vi "BLM Control Text Out.vi"(1 "BLM Control":T2={"extra wait"=0, "Stepper Value"=1e-09, "Value 1"=1.0, "Value 2"=1.0, "String 1"="", "String 2"=""} {"Value 2" format="%#_6e"; "Value 1" format="%<%H:%M:%S>t"; "extra wait" min=0; "Stepper Value" step=0.045 format="%#.7e"}) -> (0 "Command text":string[][](array[string]))   [LabVIEW 2021]
uses:
  BLM Control.ctl
panel:
  out "Est Time (H:M:S)":dbl
  out "Top or Bottom":T1(ring)
  out "String Cluster":T3
  # "BLM (Brushless Motor) Control"
  # "(BLM_ManualControl.vi needs to be open before using this program)"
  # "Distance:"
  # "deg of BLM:"
  # "seconds"
  # "AND wait extra"
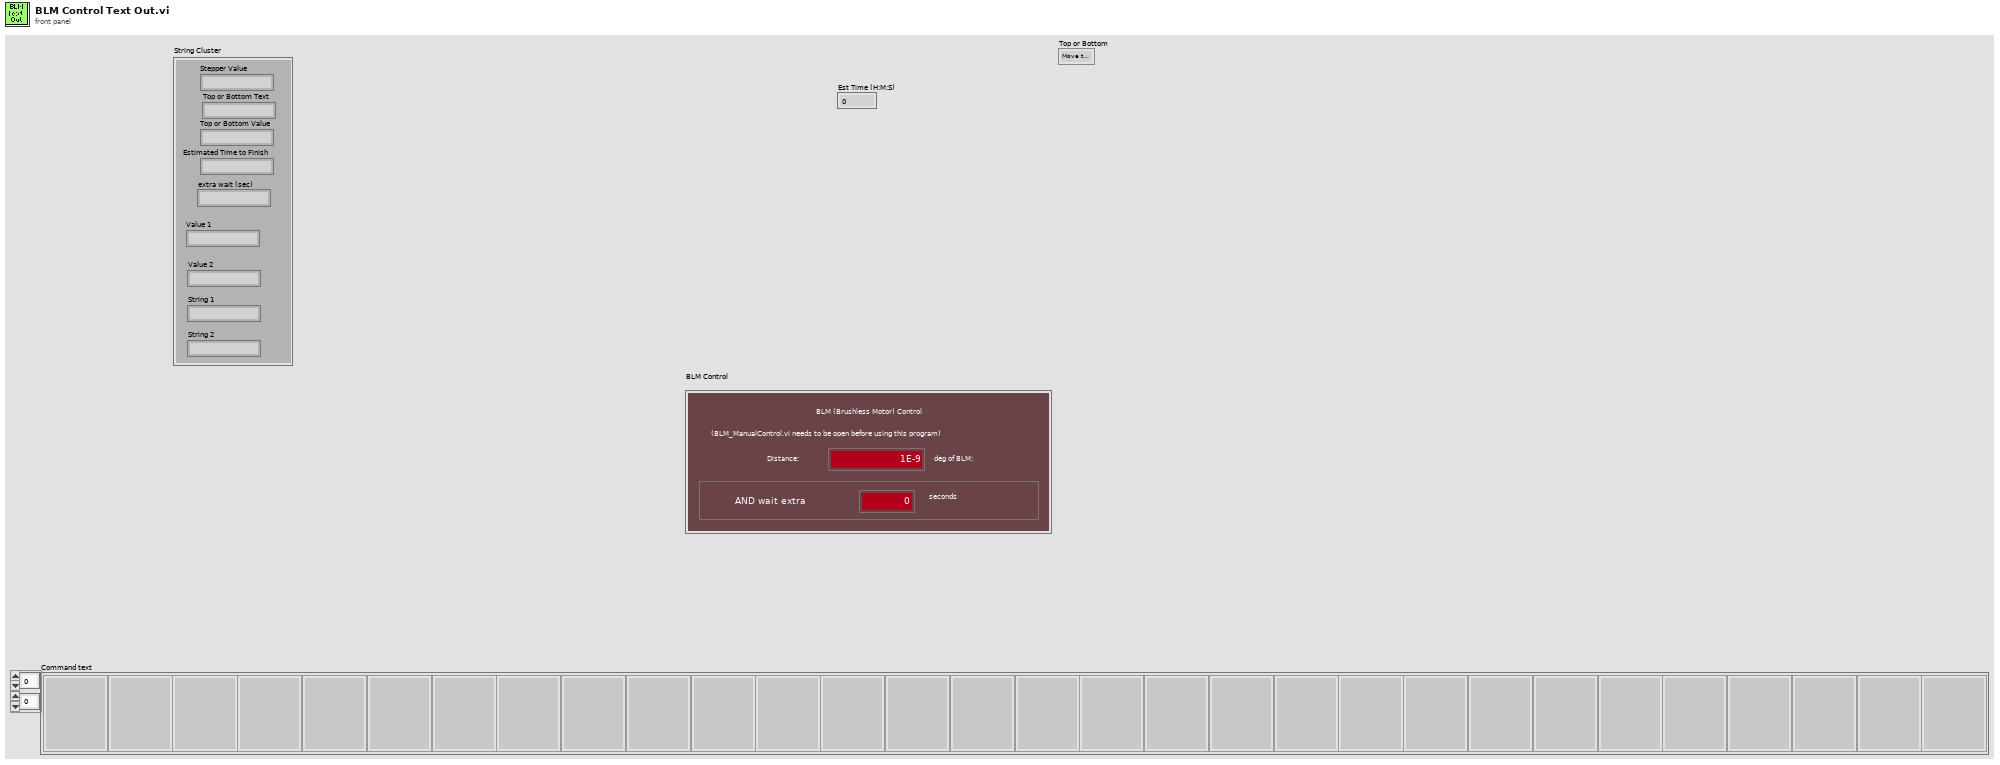
[diagram p1: front panel]
types:
  T1 = enum32{"Move to Top Position (deg)", "Move to Bottom Position (deg or in)"}
  T2 = typedef "BLM Control.ctl" = cluster{"extra wait":i32, "Stepper Value":dbl, "Value 1":dbl, "Value 2":dbl, "String 1":string, "String 2":string}
  T3 = cluster{"Stepper Value":string, "Top or Bottom Value":string, "Estimated Time to Finish":string, "extra wait (sec)":string, "Top or Bottom Text":string, "Value 1":string, "Value 2":string, "String 1":string, "String 2":string}
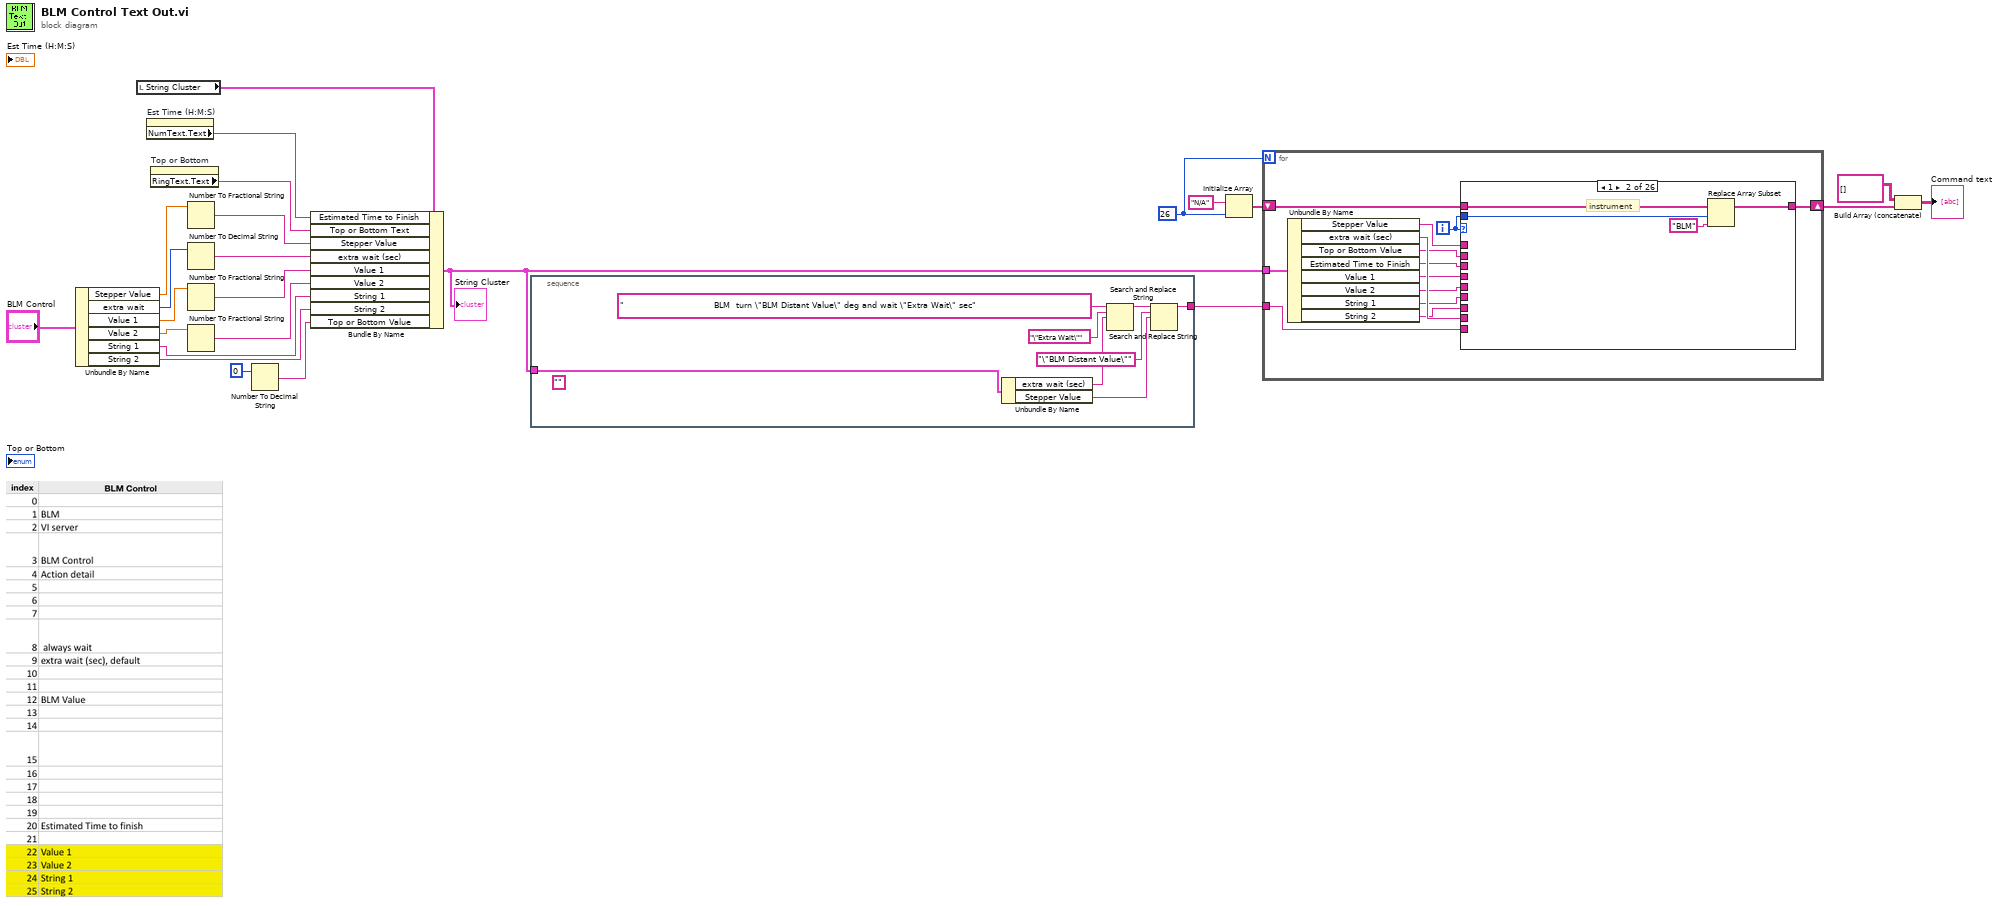
[diagram p0: block diagram]
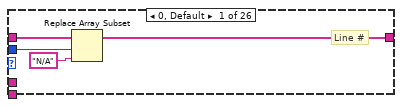
[diagram p2: hidden frame]
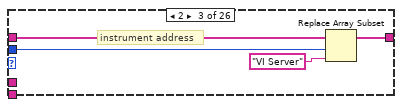
[diagram p3: hidden frame]
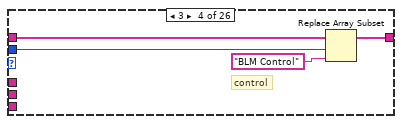
[diagram p4: hidden frame]
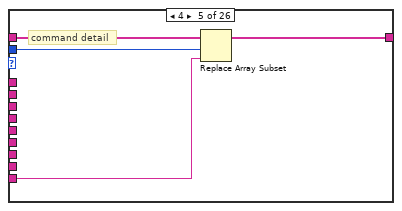
[diagram p5: hidden frame]
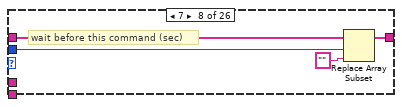
[diagram p8: hidden frame]
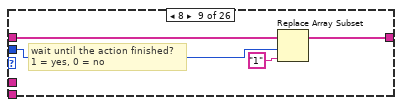
[diagram p9: hidden frame]
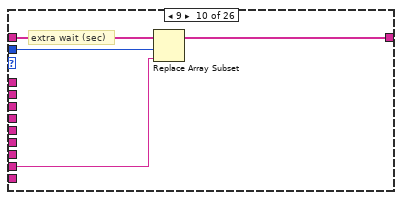
[diagram p10: hidden frame]
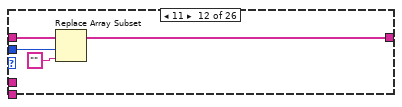
[diagram p12: hidden frame]
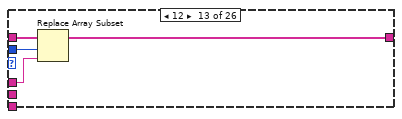
[diagram p13: hidden frame]
diagram:
  w21 = 26
  n1 = Unbundle By Name("BLM Control") -> ("Stepper Value"=w5:dbl, "extra wait"=w14:i32, "Value 1"=w12:dbl, "Value 2"=w11:dbl, "String 1"=w8:string, "String 2"=w7:string)
  n2 = local read "String Cluster"() -> (w18:T3)
  n3 = property on="Est Time (H:M:S)" class="DigNum (strict)"() -> ("NumText.Text"=w3:string)  [unwired: 2 in, 2 out]
  n4 = property on="Top or Bottom" class="Enum (strict)"() -> ("RingText.Text"=w6:string)  [unwired: 2 in, 2 out]
  n5 = Number To Fractional String(number=w5) -> (F-format string=w4:string)  [unwired: 3 in]
  n6 = Number To Decimal String(number=w14) -> (decimal integer string=w13:string)  [unwired: 1 in]
  n7 = Number To Fractional String(number=w12) -> (F-format string=w10:string)  [unwired: 3 in]
  n8 = Number To Fractional String(number=w11) -> (F-format string=w9:string)  [unwired: 3 in]
  n9 = Number To Decimal String(number=0) -> (decimal integer string=w2:string)  [unwired: 1 in]
  n10 = Bundle By Name(cluster=w18, "Estimated Time to Finish"=w3, "Top or Bottom Text"=w6, "Stepper Value"=w4, "extra wait (sec)"=w13, "Value 1"=w10, "Value 2"=w9, "String 1"=w8, "String 2"=w7, "Top or Bottom Value"=w2) -> (w16:T3)
  "String Cluster" <- w16
  n11 = stacked-sequence {
    tunnel: [w25] -> w17
    tunnel: w16 -> [w28]
    frame #0 {
      (unwired) "" ("search string")
      n12 = Unbundle By Name(w28) -> ("extra wait (sec)"=w27:string, "Stepper Value"=w26:string)
      n13 = Search and Replace String(input string="                              BLM  turn \"BLM Distant Value\" deg and wait \"Extra Wait\" sec", search string="\"Extra Wait\"", replace string=w27) -> (result string=w32:string)  [unwired: 5 in, 3 out]
      n14 = Search and Replace String(input string=w32, search string="\"BLM Distant Value\"", replace string=w26) -> (result string=w25:string)  [unwired: 5 in, 3 out]
    }
  }
  n15 = Initialize Array("N/A", w21) -> (w20:string[])
  n16 = for {
    N: w21 -> [_]
    shift-right: [w43] -> w19
    shift-left: w20 -> [w44]
    tunnel: w17 -> [w42]
    tunnel: w16 -> [w41]
    i -> [w45]
    n17 = Unbundle By Name(w41) -> ("Stepper Value"=w40:string, "extra wait (sec)"=w39:string, "Top or Bottom Value"=w34:string, "Estimated Time to Finish"=w33:string, "Value 1"=w38:string, "Value 2"=w37:string, "String 1"=w36:string, "String 2"=w35:string)
    n18 = case shown="1" w45 {
      tunnel: w45 -> [w48 w52 w57 w59 w64 _ _ w69 w73 w77 _ w82 w86 _ _ _ _ _ _ _ w97 _ w101 w106 w110 w114]
      tunnel: w44 -> [w49 w51 w56 w60 w65 w66 w67 w71 w75 w79 w80 w83 w88 w89 w90 w91 w92 w93 w94 w95 w99 w100 w103 w108 w112 w115]
      tunnel: [w46 w50 w55 w58 w63 w66 w67 w70 w74 w78 w80 w84 w87 w89 w90 w91 w92 w93 w94 w95 w98 w100 w102 w107 w111 w116] -> w43
      tunnel: w42 -> [_ _ _ _ w62 _ _ _ _ _ _ _ _ _ _ _ _ _ _ _ _ _ _ _ _ _]
      tunnel: w40 -> [_ _ _ _ _ _ _ _ _ _ _ _ w85 _ _ _ _ _ _ _ _ _ _ _ _ _]
      tunnel: w39 -> [_ _ _ _ _ _ _ _ _ w76 _ _ _ _ _ _ _ _ _ _ _ _ _ _ _ _]
      tunnel: w38 -> [_ _ _ _ _ _ _ _ _ _ _ _ _ _ _ _ _ _ _ _ _ _ w104 _ _ _]
      tunnel: w37 -> [_ _ _ _ _ _ _ _ _ _ _ _ _ _ _ _ _ _ _ _ _ _ _ w105 _ _]
      tunnel: w36 -> [_ _ _ _ _ _ _ _ _ _ _ _ _ _ _ _ _ _ _ _ _ _ _ _ w109 _]
      tunnel: w35 -> [_ _ _ _ _ _ _ _ _ _ _ _ _ _ _ _ _ _ _ _ _ _ _ _ _ w113]
      tunnel: w34 -> [_ _ _ _ _ _ _ _ _ _ _ _ _ _ _ _ _ _ _ _ _ _ _ _ _ _]
      tunnel: w33 -> [_ _ _ _ _ _ _ _ _ _ _ _ _ _ _ _ _ _ _ _ w96 _ _ _ _ _]
      frame 0, Default {
        # "Line #"
        n19 = Replace Array Subset(array=w49, new element="N/A", index=w48) -> (w46:string[])
      }
      frame 1 {
        # "instrument"
        n20 = Replace Array Subset(array=w51, new element="BLM", index=w52) -> (w50:string[])
      }
      frame 2 {
        # "instrument address"
        n21 = Replace Array Subset(array=w56, new element="VI Server" ("new element/subarray"), index=w57) -> (w55:string[])
      }
      frame 3 {
        # "control"
        n22 = Replace Array Subset(array=w60, new element="BLM Control", index=w59) -> (w58:string[])
      }
      frame 4 {
        # "command detail"
        n23 = Replace Array Subset(array=w65, new element=w62, index=w64) -> (w63:string[])
      }
      frame 5 {
        # "in  case 1"
      }
      frame 6 {
        # "in case 2"
      }
      frame 7 {
        # "wait before this command (sec)"
        n24 = Replace Array Subset(array=w71, new element="" ("new element/subarray"), index=w69) -> (w70:string[])
      }
      frame 8 {
        # "wait until the action finished?\n1 = yes, 0 = no"
        n25 = Replace Array Subset(array=w75, new element="1", index=w73) -> (w74:string[])
      }
      frame 9 {
        # "extra wait (sec)"
        n26 = Replace Array Subset(array=w79, new element=w76, index=w77) -> (w78:string[])
      }
      frame 10 {
      }
      frame 11 {
        n27 = Replace Array Subset(array=w83, new element="" ("new element/subarray"), index=w82) -> (w84:string[])
      }
      frame 12 {
        n28 = Replace Array Subset(array=w88, new element=w85, index=w86) -> (w87:string[])
      }
      frame 13 {
      }
      frame 14 {
      }
      frame 15 {
      }
      frame 16 {
      }
      frame 17 {
      }
      frame 18 {
      }
      frame 19 {
      }
      frame 20 {
        n29 = Replace Array Subset(array=w99, new element=w96, index=w97) -> (w98:string[])
      }
      frame 21 {
      }
      frame 22 {
        n30 = Replace Array Subset(array=w103, new element=w104, index=w101) -> (w102:string[])
      }
      frame 23 {
        n31 = Replace Array Subset(array=w108, new element=w105, index=w106) -> (w107:string[])
      }
      frame 24 {
        n32 = Replace Array Subset(array=w112, new element=w109, index=w110) -> (w111:string[])
      }
      frame 25 {
        n33 = Replace Array Subset(array=w115, new element=w113, index=w114) -> (w116:string[])
      }
    }
  }
  n34 = Build Array (concatenate)(string[][] [], w19) -> (→"Command text":string[][])
